vi "Keith 7001 OpenClose Chan.vi"(0 "GPIB address":string="7", 1 "error in":T1, 2 "open/close (open all:0)":u16(ring) items=["open all channels", "open channels in channel list", "close channels in channel list"], 3 "channel list":T2(array[cluster]) {"column" min=1; "channel/row" min=1; "slot/memory" min=1 max=2}) -> (4 "error out":T1)   [LabVIEW 2009, in "keithly1.lvlib"]
doc: "This VI for the Keithley 7001 Switch System allows the operator to open and close channels.\n If you try to close a forbidden channel, a device dependent error will be generated."
uses:
  keithley/keithly1.lvlib
panel:
  # "memory location\nstandard channel"
  # "matrix card\nnon-matrix card"
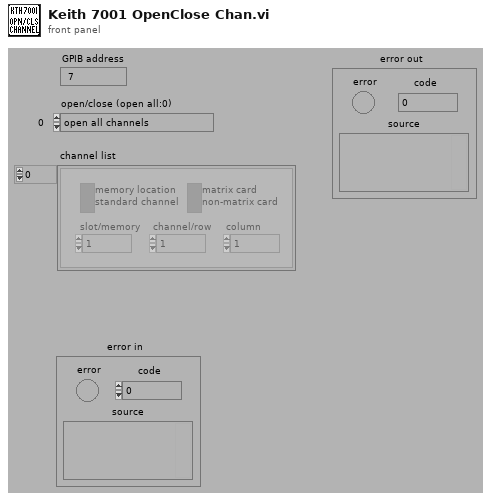
[diagram p1: front panel]
types:
  T1 = cluster{"error":bool, "code":i32, "source":string}
  T2 = cluster{"slot/memory":i16, "channel/row":i16, "column":i16, bool, bool}[]
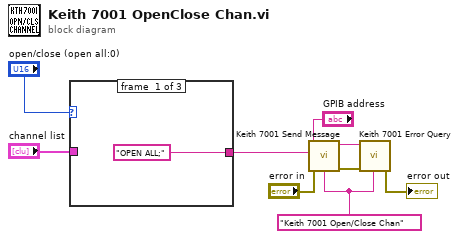
[diagram p0: block diagram]
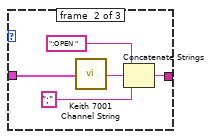
[diagram p2: hidden frame]
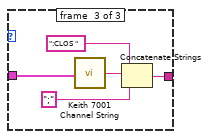
[diagram p3: hidden frame]
diagram:
  w1 = "Keith 7001 Open/Close Chan"
  n1 = case shown="2.." "open/close (open all:0)" {
    tunnel: "channel list" -> [_ w11 w17]
    tunnel: ["OPEN ALL;" w13 w18] -> w7
    frame #0 {
    }
    frame #1 {
      n2 = call "Keith 7001 Channel String.vi"("channel list"=w11) -> (0:w12:string)  [unwired: 1 in]
      n3 = Concatenate Strings(":OPEN ", w12, ";") -> (w13:string)
    }
    frame #2 {
      n4 = call "Keith 7001 Channel String.vi"("channel list"=w17) -> (0:w16:string)  [unwired: 1 in]
      n5 = Concatenate Strings(":CLOS ", w16, ";") -> (w18:string)
    }
  }
  n6 = call "Keith 7001 Send Message.vi"("address string"="GPIB address", "write buffer"=w7, "source"=w1, "error in"="error in") -> ("address out"=w4:string, "error out"=w3:T1)  [unwired: 2 in, 2 out]
  n7 = call "Keith 7001 Error Query.vi"("GPIB address"=w4, "error in"=w3, "source"=w1) -> ("error out"=→"error out":T1)  [unwired: 2 out]
